vi "libssh2_knownhost_readfile - invalid file - returns error.vi"() -> ()   [LabVIEW 2017, in "unit_tests.lvlib"]
uses:
  unit_tests.lvlib
  libssh2/libssh2_init_default.vi
  libssh2/libssh2_session_init_ex.vi
  libssh2/libssh2.lvlib
  <vilib>/PNR/Transparent Assertions/Transparent Assertions/Transparent Assertions.lvlib
panel:
  out "error out":errorcluster
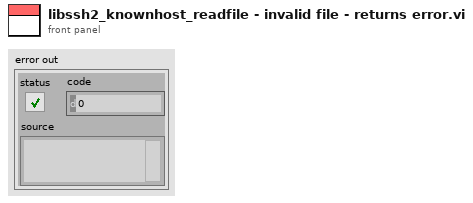
[diagram p1: front panel]
types:
  T1 = typedef "libssh2.lvlib/Session Refnum.ctl" = refnum<k1>
  T2 = typedef "libssh2.lvlib/Host Key Database Refnum.ctl" = refnum<k1>
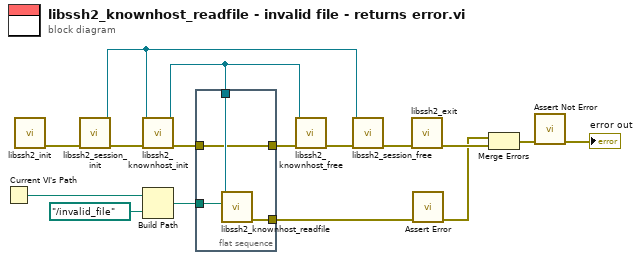
[diagram p0: block diagram]
diagram:
  n1 = Current VI's Path() -> (path=w8:path)
  n2 = call-poly "libssh2_init.vi"() -> ("error out"=w15:errorcluster)  [unwired: 11 in]
  n3 = call "libssh2_session_init.vi"("error in (no error)"=w15) -> ("error out"=w14:errorcluster, "session"=w11:T1)  [unwired: 9 in]
  n4 = call "libssh2_knownhost_init.vi"("error in (no error)"=w14, "session"=w11) -> ("error out"=w5:errorcluster, "host key database"=w9:T2)  [unwired: 8 in]
  n5 = Build Path(base path=w8, name or relative path=path "../invalid_file" ("filename")) -> (appended path=w6:path)
  n6 = flat-sequence {
    tunnel: w9 -> [w20]
    tunnel: w6 -> [w19]
    tunnel: [w18] -> w3
    tunnel: w5 -> [w17]
    tunnel: [w17] -> w4
    frame #0 {
      n7 = call "libssh2_knownhost_readfile.vi"("filename"=w19, "host key database"=w20) -> ("error out"=w18:errorcluster)  [unwired: 8 in, 1 out]
    }
  }
  n8 = call "libssh2_knownhost_free.vi"("error in (no error)"=w4, "host key database"=w9) -> ("error out"=w10:errorcluster)  [unwired: 9 in]
  n9 = call "libssh2_session_free.vi"("error in (no error)"=w10, "session"=w11) -> ("error out"=w13:errorcluster)  [unwired: 9 in]
  n10 = call "libssh2_exit.vi"("error in (no error)"=w13) -> ("error out"=w12:errorcluster)  [unwired: 10 in]
  n11 = call <vilib>:"Assert Error.vi"("error in (no error)"=w3) -> ("error out"=w1:errorcluster)  [unwired: 10 in]
  n12 = Merge Errors(w1, w12) -> (w2:errorcluster)
  n13 = call <vilib>:"Assert Not Error.vi"("error in (no error)"=w2) -> ("error out"=→"error out":errorcluster)  [unwired: 10 in]
